vi "Apply Graph Preferences.vi"(5 "Auto Scale":bool, 6 "Graph Ref":refnum<vi>, 7 "Overlay Data":cluster{"X":sgl[], "Y":sgl[]}, 9 "Log Scale":bool, 10 "CPS":bool, 11 "Averaging":bool) -> ()   [LabVIEW 2015]
panel:
  in  "Dwell Time (mS)":dbl
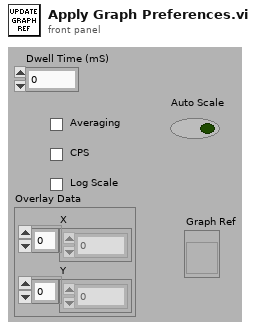
[diagram p1: front panel]
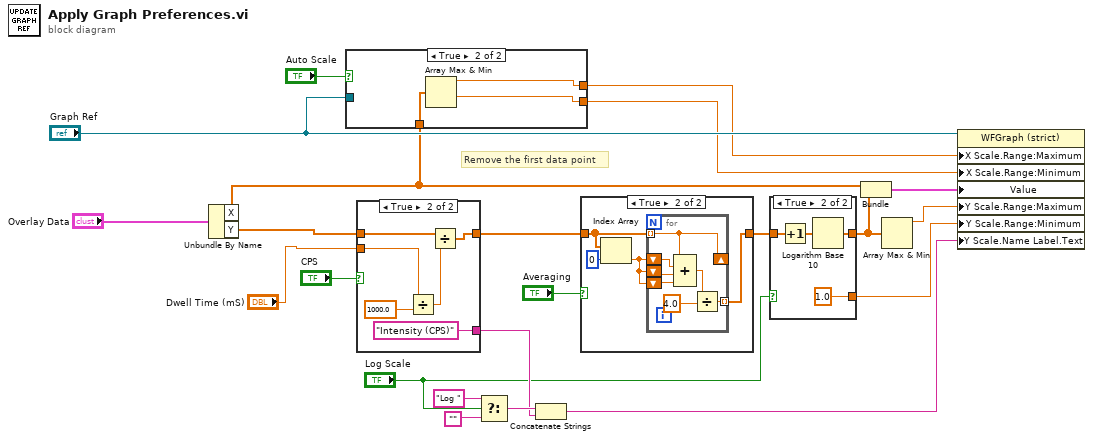
[diagram p0: block diagram]
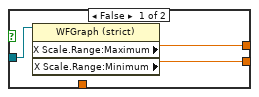
[diagram p2: hidden frame]
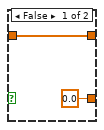
[diagram p3: hidden frame]
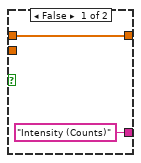
[diagram p5: hidden frame]
diagram:
  # "Remove the first data point"
  n1 = Unbundle By Name("Overlay Data") -> ("X"=w4:sgl[], "Y"=w3:sgl[])
  n2 = case shown="True" "Auto Scale" {
    tunnel: w4 -> [_ w28]
    tunnel: [w24 w26] -> w10
    tunnel: [w25 w27] -> w9
    tunnel: "Graph Ref" -> [w23 _]
    frame False {
      n3 = property class="WFGraph (strict)"(reference=w23) -> ("X Scale.Range:Maximum"=w25:dbl, "X Scale.Range:Minimum"=w24:dbl)  [unwired: 1 in, 2 out]
    }
    frame True {
      n4 = Array Max & Min(array=w28) -> (max value=w27:sgl, min value=w26:sgl)  [unwired: 2 out]
    }
  }
  n5 = case shown="True" "CPS" {
    tunnel: w3 -> [w30 w35]
    tunnel: [w30 w33] -> w5
    tunnel: ["Intensity (Counts)" "Intensity (CPS)"] -> w16
    tunnel: "Dwell Time (mS)" -> [_ w31]
    frame False {
    }
    frame True {
      n6 = Divide(x=w31, y=1000.0) -> (x/y=w34:dbl)
      n7 = Divide(x=w35, y=w34) -> (x/y=w33:dbl[])
    }
  }
  n8 = Select(t="Log ", s="Log Scale", f="") -> (s? t:f=w17:string)
  n9 = Concatenate Strings(w17, w16) -> (w11:string)
  n10 = case shown="True" "Averaging" {
    tunnel: w5 -> [w37 w39]
    tunnel: [w37 w38] -> w15
    frame False {
    }
    frame True {
      n11 = Index Array(array=w39, index=0) -> (element=w40:dbl)
      n12 = for {
        shift-right: [w45] -> _
        shift-left: w40 -> [w48]
        shift-left: w40 -> [w47]
        shift-left: w40 -> [w46]
        tunnel: w39 -> [w45] mode=indexing
        tunnel: [w42] -> w38 mode=indexing
        n13 = Compound Arithmetic op=ADD(w45, w48, w47, w46) -> (w44:dbl)
        n14 = Divide(x=w44, y=4.0) -> (x/y=w42:dbl)
      }
    }
  }
  n15 = case shown="True" "Log Scale" {
    tunnel: w15 -> [w50 w54]
    tunnel: [w50 w53] -> w14
    tunnel: [0.0 ("y") 1.0 ("y")] -> w8
    frame False {
    }
    frame True {
      n16 = Increment(x=w54) -> (x+1=w51:dbl[])
      n17 = Logarithm Base 10(1:w51) -> (0:w53:dbl[])
    }
  }
  n18 = Bundle("X"=w4, "Y"=w14) -> (w12:cluster{"X":sgl[], "Y":dbl[]})  [unwired: 1 out]
  n19 = Array Max & Min(array=w14) -> (max value=w7:dbl)  [unwired: 3 out]
  n20 = property class="WFGraph (strict)"(reference="Graph Ref", "X Scale.Range:Maximum"=w9, "X Scale.Range:Minimum"=w10, "Value"=w12, "Y Scale.Range:Maximum"=w7, "Y Scale.Range:Minimum"=w8, "Y Scale.Name Label.Text"=w11) -> ()  [unwired: 1 in, 2 out]
